vi "Write Firmware Version.vi"(8 "Setup.Firmware Valid":bool, 9 "Setup.Firmware Minor":u16, 10 "Setup.Firmware Major":u16, 11 "DCM - RT in":refnum<class "DCM - RT.lvclass">) -> (3 "DCM - RT out":refnum<class "DCM - RT.lvclass">)   [LabVIEW 2016, in "DCM-Classes.lvlib" / "DCM - RT.lvclass"]
uses:
  DCM - RT.lvclass
  DCM - RT.lvclass/DCM - RT.ctl
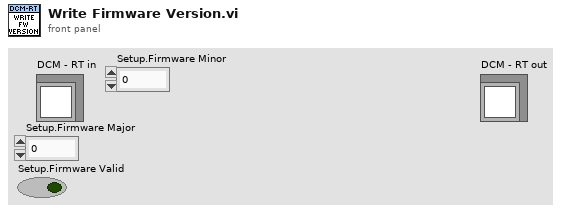
[diagram p1: front panel]
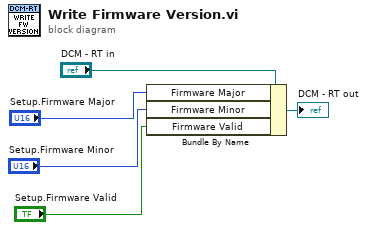
[diagram p0: block diagram]
diagram:
  n1 = Bundle By Name(cluster="DCM - RT in", "Firmware Major"="Setup.Firmware Major", "Firmware Minor"="Setup.Firmware Minor", "Firmware Valid"="Setup.Firmware Valid") -> (→"DCM - RT out":refnum<class "DCM - RT.lvclass">)
